vi "FRIC_navX_Get_RawValues_GyroAccelMag.vi"(7 "Update":bool) -> (2 "Raw Values (out)":T1)   [LabVIEW 2015, in "navX AE v1.lvlib"]
doc: "This navX VI returns the raw values from the Gyro, Accel, and Mag sensors."
uses:
  navX AE v1.lvlib
  navX Library v2/_TypeDefs/Z900_navX_DeviceRegisters.ctl
  navX Library v2/navX Library v2.lvlib
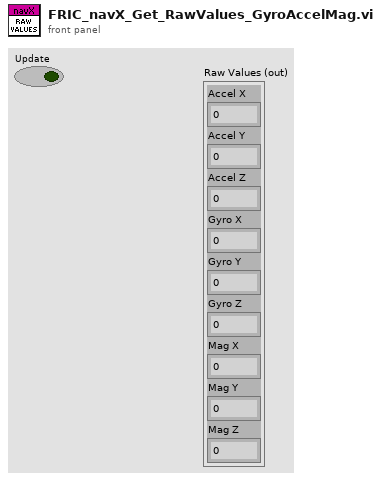
[diagram p1: front panel]
types:
  T1 = cluster{"Accel X":dbl, "Accel Y":dbl, "Accel Z":dbl, "Gyro X":dbl, "Gyro Y":dbl, "Gyro Z":dbl, "Mag X":dbl, "Mag Y":dbl, "Mag Z":dbl}
  T2 = typedef "navX Library v2.lvlib/Z900_navX_DeviceRegisters.ctl" = u8
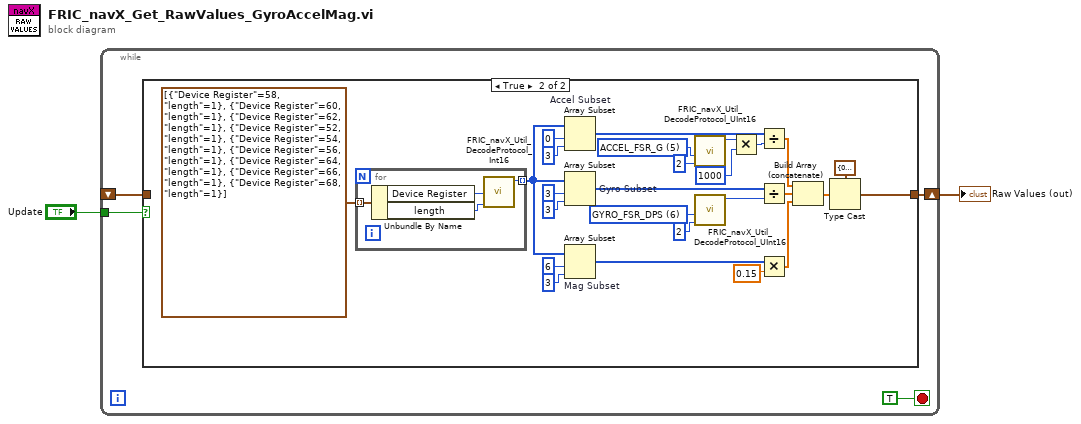
[diagram p0: block diagram]
diagram:
  n1 = while {
    shift-right: [w6] -> w2
    shift-left: _ -> [w3]
    tunnel: "Update" -> [w4]
    stop <- TRUE stop-if-true
    n2 = case shown="True" w4 {
      tunnel: [w7 w33] -> w6
      tunnel: w3 -> [w7 _]
      frame False {
      }
      frame True {
        w11 = T2 5 items=["WHOAMI"=0, "HW_REV"=1, "FW_VER_MAJOR"=2, "FW_VER_MINOR"=3, "UPDATE_RATE_HZ"=4, "ACCEL_FSR_G"=5, "GYRO_FSR_DPS"=6, "OP_STATUS"=8, "CAL_STATUS"=9, "SELFTEST_STATUS"=10, "CAPABILITY_FLAGS_L"=11, "CAPABILITY_FLAGS_H"=12, "SENSOR_STATUS"=16, "TIMESTAMP"=18, "YAW"=22, "ROLL"=24, "PITCH"=26, "HEADING"=28, "FUSED_HEADING"=30, "ALTITUDE_I"=32, "ALTITUDE_D"=34, "LINERA_ACC_X"=36, "LINERA_ACC_Y"=38, "LINERA_ACC_Z"=40, "QUAT_W"=42, "QUAT_X"=44, "QUAT_Y"=46, "QUAT_Z"=48, "MPU_TEMP_C"=50, "GYRO_X"=52, "GYRO_Y"=54, "GYRO_Z"=56, "ACC_X"=58, "ACC_Y"=60, "ACC_Z"=62, "MAG_X"=64, "MAG_Y"=66, "MAG_Z"=68, "PRESSURE_I"=70, "PRESSURE_D"=72, "PRESSURE_TEMP"=74, "YAW_OFFSET"=76, "QUAT_OFFSET_W"=78, "QUAT_OFFSET_X"=80, "QUAT_OFFSET_Y"=82, "QUAT_OFFSET_Z"=84, "INTEGRATION_CONTROL"=86, "VELOCITY_X"=88, "VELOCITY_Y"=92, "VELOCITY_Z"=96, "DISPLACMENT_X"=100, "DISPLACMENT_Y"=104, "DISPLACEMENT_Z"=108] ("Device Register")
        w15 = T2 6 items=["WHOAMI"=0, "HW_REV"=1, "FW_VER_MAJOR"=2, "FW_VER_MINOR"=3, "UPDATE_RATE_HZ"=4, "ACCEL_FSR_G"=5, "GYRO_FSR_DPS"=6, "OP_STATUS"=8, "CAL_STATUS"=9, "SELFTEST_STATUS"=10, "CAPABILITY_FLAGS_L"=11, "CAPABILITY_FLAGS_H"=12, "SENSOR_STATUS"=16, "TIMESTAMP"=18, "YAW"=22, "ROLL"=24, "PITCH"=26, "HEADING"=28, "FUSED_HEADING"=30, "ALTITUDE_I"=32, "ALTITUDE_D"=34, "LINERA_ACC_X"=36, "LINERA_ACC_Y"=38, "LINERA_ACC_Z"=40, "QUAT_W"=42, "QUAT_X"=44, "QUAT_Y"=46, "QUAT_Z"=48, "MPU_TEMP_C"=50, "GYRO_X"=52, "GYRO_Y"=54, "GYRO_Z"=56, "ACC_X"=58, "ACC_Y"=60, "ACC_Z"=62, "MAG_X"=64, "MAG_Y"=66, "MAG_Z"=68, "PRESSURE_I"=70, "PRESSURE_D"=72, "PRESSURE_TEMP"=74, "YAW_OFFSET"=76, "QUAT_OFFSET_W"=78, "QUAT_OFFSET_X"=80, "QUAT_OFFSET_Y"=82, "QUAT_OFFSET_Z"=84, "INTEGRATION_CONTROL"=86, "VELOCITY_X"=88, "VELOCITY_Y"=92, "VELOCITY_Z"=96, "DISPLACMENT_X"=100, "DISPLACMENT_Y"=104, "DISPLACEMENT_Z"=108] ("Device Register")
        n3 = for {
          tunnel: cluster{"Device Register":T2, "length":i32}[] [{"Device Register"=58, "length"=1}, {"Device Register"=60, "length"=1}, {"Device Register"=62, "length"=1}, {"Device Register"=52, "length"=1}, {"Device Register"=54, "length"=1}, {"Device Register"=56, "length"=1}, {"Device Register"=64, "length"=1}, {"Device Register"=66, "length"=1}, {"Device Register"=68, "length"=1}] ("Array") -> [w35] mode=indexing
          tunnel: [w34] -> w8 mode=indexing
          n4 = Unbundle By Name(w35) -> ("Device Register"=w37:T2, "length"=w36:i32)
          n5 = call "FRIC_navX_Util_DecodeProtocol_Int16.vi"("length"=w36, "Device Register"=w37) -> ("Value"=w34:i16)  [unwired: 9 in]
        }
        n6 = Array Subset "Accel Subset"(array=w8, index=0, length=3) -> (w26:i16[])
        n7 = Array Subset "Gyro Subset"(array=w8, index=3, length=3) -> (w25:i16[])
        n8 = Array Subset "Mag Subset"(array=w8, index=6, length=3) -> (w23:i16[])
        n9 = call "FRIC_navX_Util_DecodeProtocol_UInt16.vi"("length"=2, "Device Register"=w11) -> ("Value"=w9:u16)  [unwired: 9 in]
        n10 = call "FRIC_navX_Util_DecodeProtocol_UInt16.vi"("length"=2, "Device Register"=w15) -> ("Value"=w13:u16)  [unwired: 9 in]
        n11 = Multiply(x=w9, y=u16 1000) -> (x*y=w16:u16)
        n12 = Divide(x=w26, y=w16) -> (x/y=w22:dbl[])
        n13 = Divide(x=w25, y=w13) -> (x/y=w21:dbl[])
        n14 = Multiply(x=w23, y=0.15) -> (x*y=w20:dbl[])
        n15 = Build Array (concatenate)(w22, w21, w20) -> (w19:dbl[])
        n16 = Type Cast(type=T1 {"Accel X"=0.0, "Accel Y"=0.0, "Accel Z"=0.0, "Gyro X"=0.0, "Gyro Y"=0.0, "Gyro Z"=0.0, "Mag X"=0.0, "Mag Y"=0.0, "Mag Z"=0.0}, x=w19) -> (*(type *) &x=w33:T1)
      }
    }
  }
  "Raw Values (out)" <- w2
